vi "Write Timestamp Type.vi"(8 "error in (no error)":errorcluster, 10 "timestamp type":T1=1 caption="timestamp Type (absolute)" items=["relative", "absolute"], 11 "PXIe5105 in":refnum<class "PXIe5105.lvclass">) -> (0 "error out":errorcluster, 3 "PXIe5105 out":refnum<class "PXIe5105.lvclass">)   [LabVIEW 2018, in "PXIe5105.lvlib" / "PXIe5105.lvclass"]
uses:
  PXIe5105.lvclass
  <instrlib>/niScope/Controls/niScope timestamp type.ctl
  PXIe5105.lvclass/PXIe5105.ctl
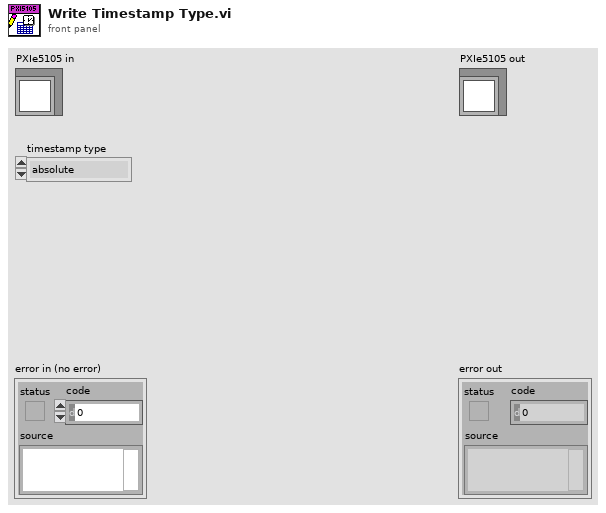
[diagram p1: front panel]
types:
  T1 = typedef "niScope timestamp type.ctl" = i32
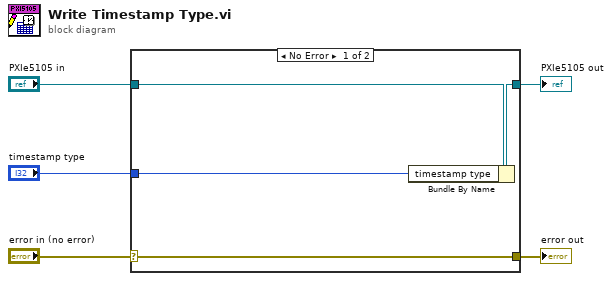
[diagram p0: block diagram]
diagram:
  n1 = case shown="No Error" "error in (no error)" {
    selector: "error in (no error)" -> [w9 w10]
    tunnel: [w9 w10] -> w4
    tunnel: [w7 w11] -> w2
    tunnel: "PXIe5105 in" -> [w8 w11]
    tunnel: "timestamp type" -> [w6 _]
    frame No Error {
      n2 = Bundle By Name(cluster=w8, "timestamp type"=w6) -> (w7:refnum<class "PXIe5105.lvclass">)
    }
    frame Error {
    }
  }
  "error out" <- w4
  "PXIe5105 out" <- w2
